vi "LWXPS_GroupAnalogTrackingModeEnable.vi"(6 "LabVIEW error IN":errorcluster, 7 "Tracking Type":string, 8 "Group Name":string, 9 "XPS Reference IN":refnum<k24>) -> (0 "LabVIEW error OUT":errorcluster, 1 "XPS Error String":string, 2 "Returned error code":i32, 3 "XPS Reference OUT":refnum<k24>)   [LabVIEW 2015]
uses:
  C:/Users/Becky/Desktop/XPS-UNIFIED/LabVIEW VIs/LabVIEW Source Code/Dll/Newport.XPS.CommandInterface.dll
  Dll/Newport.XPS.CommandInterface.dll
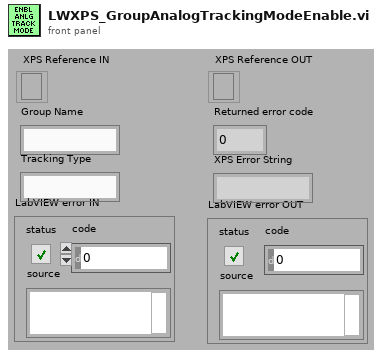
[diagram p1: front panel]
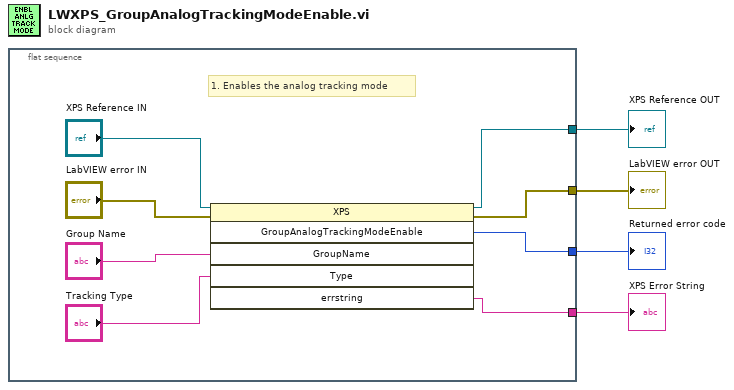
[diagram p0: block diagram]
diagram:
  n1 = flat-sequence {
    tunnel: [w9] -> w4
    tunnel: [w12] -> w3
    tunnel: [w10] -> w2
    tunnel: [w6] -> w1
    frame #0 {
      # "1. Enables the analog tracking mode"
      n2 = invoke class="XPS" method="GroupAnalogTrackingModeEnable"(reference="XPS Reference IN", error in="LabVIEW error IN", "GroupName"="Group Name", "Type"="Tracking Type") -> (reference out=w9:refnum<k24>, error out=w12:errorcluster, "GroupAnalogTrackingModeEnable"=w10:i32, "errstring"=w6:string)  [unwired: 2 in, 2 out]
    }
  }
  "XPS Reference OUT" <- w4
  "LabVIEW error OUT" <- w3
  "Returned error code" <- w2
  "XPS Error String" <- w1
